vi "Fourtrack.vi"(8 "error in (no error)":errorcluster, 9 "Track Division in Samples":i32, 10 "Track (File) References in":T2, 11 "Refnum in":T1) -> (0 "error out":errorcluster, 2 "Track (File) References out":T2, 3 "Refnum out":T1)   [LabVIEW 2014]
uses:
  Controls/FPGA Reference.ctl
  Controls/Track (File) References.ctl
  Controls/Track Enable.ctl
  Controls/Audio In.ctl
  Sub VIs/Audio/Controls/playback state.ctl
  Controls/Application Data.vi
  <vilib>/Utility/error.llb/Error Cluster From Error Code.vi
  <vilib>/rvi/errors/niLvFpgaAdjustHostInterfaceError.vi
  Sub VIs/Audio/Controls/sample block size.vi
  <vilib>/rvi/interface/nirviReadWriteControl/nirviReadWriteControl.xnode
  NiFpgaLv.dll
  <vilib>/rvi/interface/Simulation/niFpgaSimulationCallBeginRW.vi
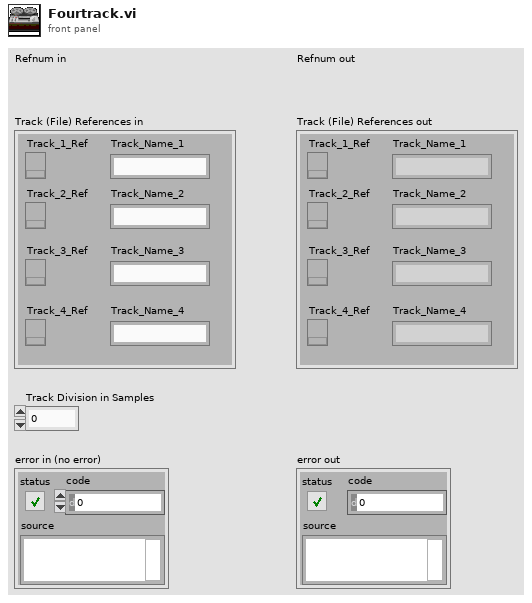
[diagram p1: front panel]
types:
  T1 = typedef "FPGA Reference.ctl" = refnum<k20>
  T2 = typedef "Track (File) References.ctl" = cluster{"Track_1_Ref":refnum<k34>, "Track_2_Ref":refnum<k34>, "Track_3_Ref":refnum<k34>, "Track_4_Ref":refnum<k34>, "Track_Name_1":string, "Track_Name_2":string, "Track_Name_3":string, "Track_Name_4":string}
  T3 = typedef "Track Controls.ctl" = cluster{"Track 0":T4, "Track 1":T4, "Track 2":T4, "Track 3":T4}
  T4 = typedef "Track Volume Settings.ctl" = cluster{"Volume":dbl, "Pan":dbl, "Record":bool, "FX":bool}
  T5 = cluster{"FX":bool, "FX":bool, "FX":bool, "FX":bool}
  T6 = typedef "Track Enable.ctl" = cluster{"Track_0 _Enable ":bool, "Track_1 _Enable ":bool, "Track_2 _Enable ":bool, "Track_3 _Enable ":bool}
  T7 = typedef "Audio In.ctl" = cluster{"AudioIn/Left (N Samples)":i16[], "AudioIn/Right (N Samples)":i16[]}
  T8 = typedef "playback state.ctl" = enum16{"Load File", "Save File", "Play", "Record", "Stop", "Rewind"}
  T9 = typedef "4 Track Audio.ctl" = cluster{"Track 0":T7, "Track 1":T7, "Track 2":T7, "Track 3":T7}
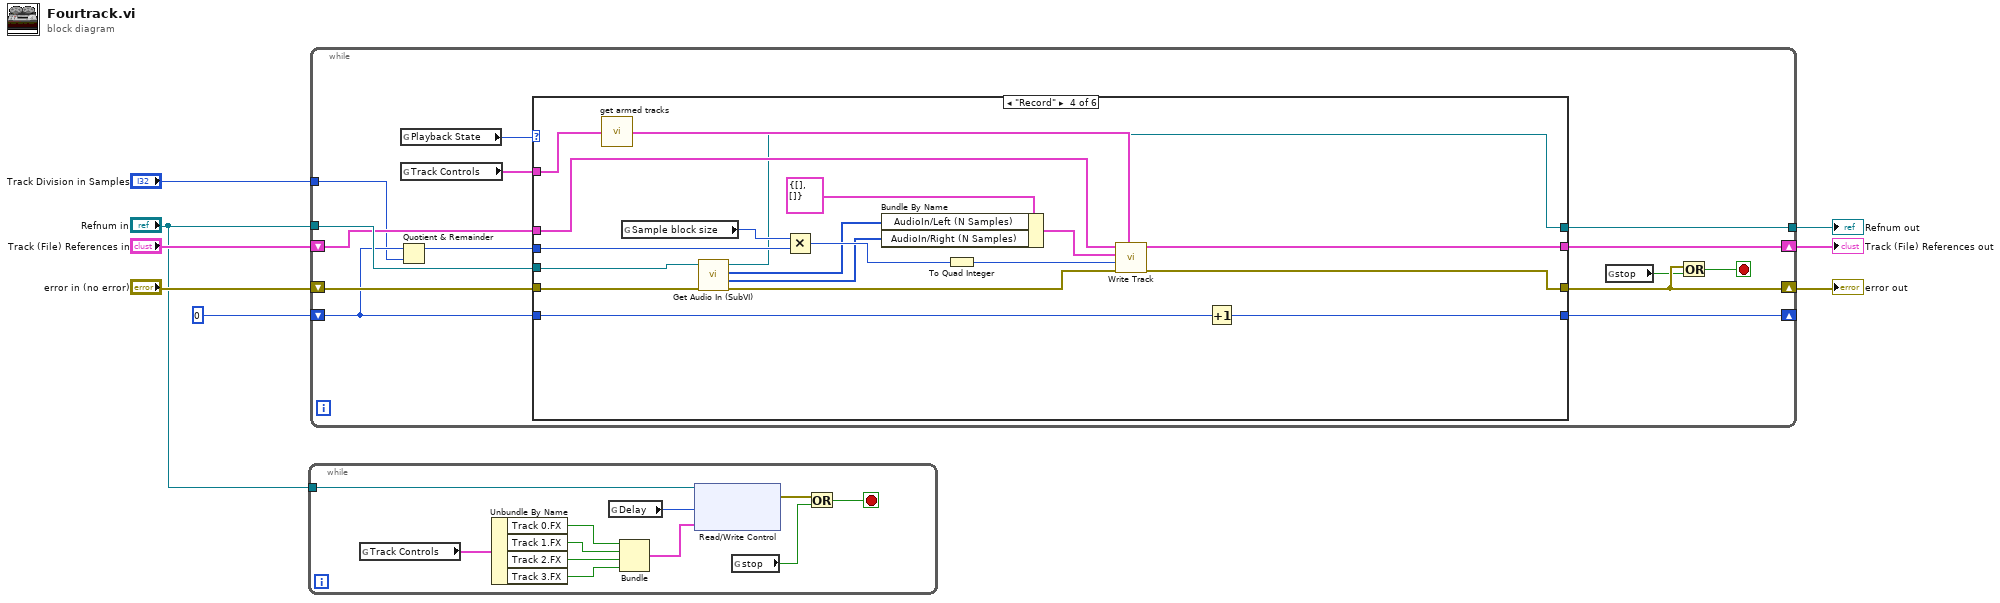
[diagram p0: block diagram]
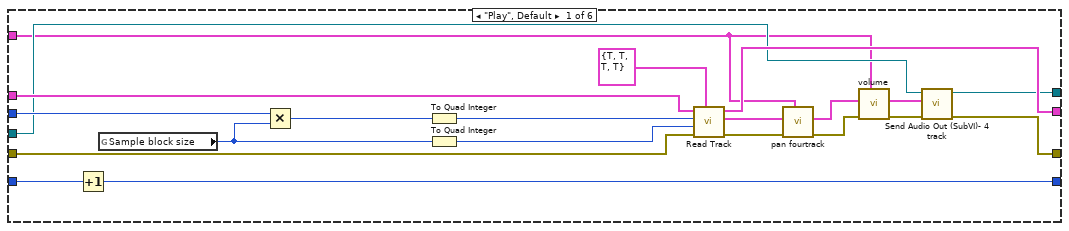
[diagram p2: hidden frame]
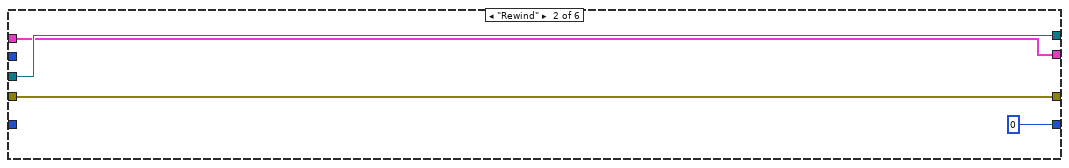
[diagram p3: hidden frame]
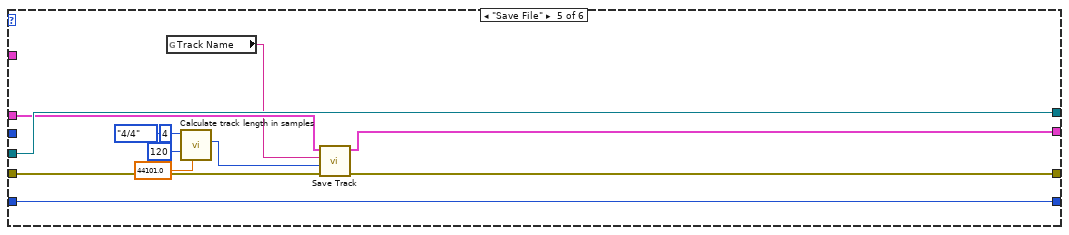
[diagram p5: hidden frame]
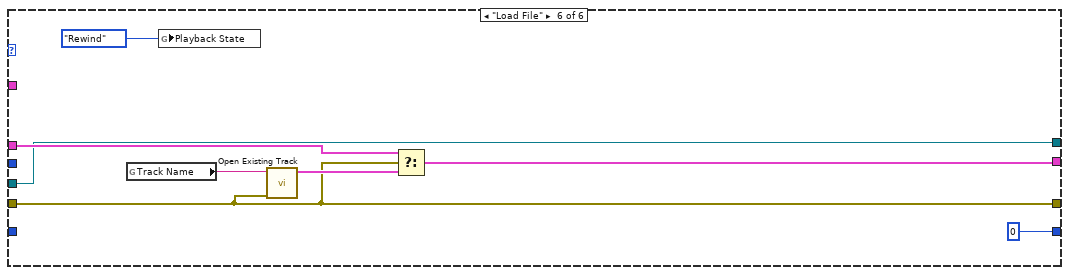
[diagram p6: hidden frame]
diagram:
  n1 = while {
    tunnel: "Refnum in" -> [w17]
    stop <- w18 stop-if-true
    n2 = global read "Application Data.vi" "Track Controls"() -> (w14:T3)
    n3 = Unbundle By Name(w14) -> ("Track 0.FX"=w12:bool, "Track 1.FX"=w13:bool, "Track 2.FX"=w11:bool, "Track 3.FX"=w10:bool)
    n4 = global read "Application Data.vi" "Delay"() -> (w15:u32)
    n5 = Bundle("FX"=w12, "FX"=w13, "FX"=w11, "FX"=w10) -> (w9:T5)  [unwired: 1 in]
    n6 = xnode "Read/Write Control"("FPGA VI Reference In"=w17, "Delay_ticks"=w15, "Delay_Enable"=w9) -> ("error out"=w16:errorcluster)  [unwired: 1 in, 1 out]
    n7 = global read "Application Data.vi" "stop"() -> (w19:bool)
    n8 = Or(x=w16, y=w19) -> (x .or. y?=w18:bool)
  }
  n9 = while {
    shift-right: [w26] -> w4
    shift-left: "Track (File) References in" -> [w27]
    shift-right: [w31] -> w8
    shift-left: "error in (no error)" -> [w32]
    shift-right: [w29] -> _
    shift-left: 0 -> [w22]
    tunnel: "Refnum in" -> [w33]
    tunnel: [w28] -> w2
    tunnel: "Track Division in Samples" -> [w21]
    stop <- w30 stop-if-true
    n10 = Quotient & Remainder(x=w22, y=w21) -> (x-y*floor(x/y)=w20:i32)  [unwired: 1 out]
    n11 = global read "Application Data.vi" "Playback State"() -> (w24:T8)
    n12 = global read "Application Data.vi" "Track Controls"() -> (w25:T3)
    n13 = case shown="\"Record\"" w24 {
      tunnel: w25 -> [w34 _ _ w67 _ _]
      tunnel: w33 -> [w39 w56 w60 w63 w92 w95]
      tunnel: w32 -> [w42 w58 w62 w71 w88 w97]
      tunnel: [w45 w58 w62 w64 w87 w97] -> w31
      tunnel: w20 -> [w53 _ w61 w77 _ _]
      tunnel: [w54 0 w61 w81 w93 0] -> w29
      tunnel: [w46 w56 w60 w66 w92 w95] -> w28
      tunnel: w27 -> [w48 w55 w59 w72 w91 w100]
      tunnel: [w47 w55 w59 w80 w89 w98] -> w26
      tunnel: w22 -> [w52 _ _ w75 w93 _]
      frame "Play", Default {
        n14 = Increment(x=w52) -> (x+1=w54:i32)
        n15 = global read "sample block size.vi" "Sample block size"() -> (w43:i32)
        n16 = Multiply(x=w53, y=w43) -> (x*y=w44:i32)
        n17 = To Quad Integer(1:w44) -> (0:w50:i64)
        n18 = To Quad Integer(1:w43) -> (0:w51:i64)
        n19 = call "Read Track.vi"("Track Enable"=T6 {"Track_0 _Enable "=TRUE, "Track_1 _Enable "=TRUE, "Track_2 _Enable "=TRUE, "Track_3 _Enable "=TRUE}, "Error In"=w42, "Number Of Elements to Read"=w51, "Read Position"=w50, "Track (File) References In"=w48) -> ("Error Out"=w38:errorcluster, "4-Track Audio"=w35:T9, "Track (File) References Out"=w47:T2)  [unwired: 4 in]
        n20 = call "pan fourtrack.vi"("Track Controls"=w34, "error in (no error)"=w38, "4-Track Audio in"=w35) -> ("error out"=w37:errorcluster, "4-Track Audio out"=w36:T9)  [unwired: 7 in]
        n21 = call "volume.vi"("Track Controls"=w34, "error in (no error)"=w37, "4-Track Audio in"=w36) -> ("error out"=w41:errorcluster, "4-Track Audio out"=w40:T9)  [unwired: 7 in]
        n22 = call "Send Audio Out (SubVI)- 4 track.vi"("error in (no error)"=w41, "4-Track Audio out"=w40, "Refnum in"=w39) -> ("error out"=w45:errorcluster, "Refnum out"=w46:T1)  [unwired: 7 in]
      }
      frame "Rewind" {
      }
      frame "Stop" {
      }
      frame "Record" {
        n23 = call "get armed tracks.vi"("Track Controls"=w67) -> ("Track Enable"=w68:T6)
        n24 = global read "sample block size.vi" "Sample block size"() -> (w70:i32)
        n25 = call "Get Audio In (SubVI).vi"("error in (no error)"=w71, "Refnum in"=w63) -> ("error out"=w78:errorcluster, "Right Audio In"=w73:i16[], "Left Audio In"=w74:i16[], "Refnum out"=w66:T1)  [unwired: 6 in]
        n26 = Multiply(x=w70, y=w77) -> (x*y=w76:i32)
        n27 = Bundle By Name(cluster=T7 {"AudioIn/Left (N Samples)"=[], "AudioIn/Right (N Samples)"=[]} ("Audio In"), "AudioIn/Left (N Samples)"=w74, "AudioIn/Right (N Samples)"=w73) -> (w65:T7)
        n28 = To Quad Integer(1:w76) -> (0:w69:i64)
        n29 = call "Write Track.vi"("Track Enable"=w68, "Error In"=w78, "Write Position"=w69, "Audio In"=w65, "Track (File) References In"=w72) -> ("Error Out"=w64:errorcluster, "Track (File) References Out"=w80:T2)  [unwired: 5 in]
        n30 = Increment(x=w75) -> (x+1=w81:i32)
      }
      frame "Save File" {
        n31 = global read "Application Data.vi" "Track Name"() -> (w90:string)
        n32 = call "Calculate track length in samples.vi"("Sample Rate (Hz)"=44101.0, "Time Signature"=enum16{"4/4", "3/4"}."4/4", "BPM"=120, "Measures"=4) -> ("Track Length in Samples"=w82:i32)  [unwired: 4 in, 3 out]
        n33 = call "Save Track.vi"("Error In"=w88, "Samples Per Channel\\File Size"=w82, "Track Name of Copy"=w90, "Track (File) References"=w91) -> ("Error Out"=w87:errorcluster, "Track (File) References Out"=w89:T2)  [unwired: 6 in]
      }
      frame "Load File" {
        n34 = global read "Application Data.vi" "Track Name"() -> (w101:string)
        n35 = global write "Application Data.vi" "Playback State"(playback_state."Rewind" ("Playback State")) -> ()
        n36 = call "Open Existing Track.vi"("error in (no error)"=w97, "Track Name"=w101) -> ("Track (File) References"=w99:T2)  [unwired: 8 in, 1 out]
        n37 = Select(t=w100, s=w97, f=w99) -> (s? t:f=w98:T2)
      }
    }
    n38 = global read "Application Data.vi" "stop"() -> (w23:bool)
    n39 = Or(x=w31, y=w23) -> (x .or. y?=w30:bool)
  }
  "error out" <- w8
  "Track (File) References out" <- w4
  "Refnum out" <- w2
